vi "Read Sorting Column.vi"(8 "error in":errorcluster, 11 "EngineTags in":refnum<class "Engine Mappings.lvclass">) -> (0 "error out":errorcluster, 2 "Sorting Column":i32, 3 "EngineTags out":refnum<class "Engine Mappings.lvclass">)   [LabVIEW 2013, in "PL Framework Configuration Tool.lvlib" / "Engine Mappings.lvclass"]
uses:
  Engine Mappings.lvclass
  Engine Mappings.lvclass/Engine Mappings.ctl
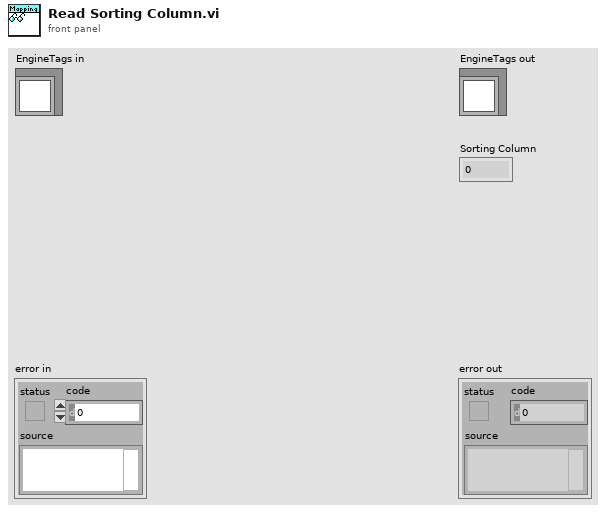
[diagram p1: front panel]
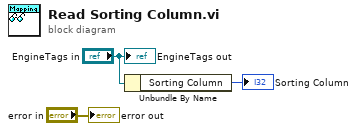
[diagram p0: block diagram]
diagram:
  n1 = Unbundle By Name("EngineTags in") -> ("Sorting Column"=→"Sorting Column":i32)
  "error out" <- "error in"
  "EngineTags out" <- "EngineTags in"
